vi "startService.vi"(8 "error in (no error)":errorcluster, 11 "M1M3SAL in":refnum<class "M1M3SAL.lvclass">) -> (0 "error out":errorcluster, 3 "M1M3SAL out":refnum<class "M1M3SAL.lvclass">)   [LabVIEW 2016, in "M1M3SupportCommunicator.lvlib" / "M1M3SAL.lvclass"]
uses:
  M1M3SAL.lvclass
  M1M3SAL.lvclass/M1M3SAL.ctl
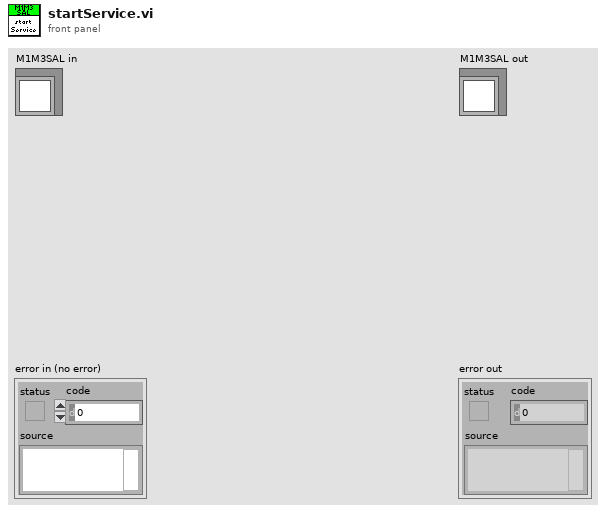
[diagram p1: front panel]
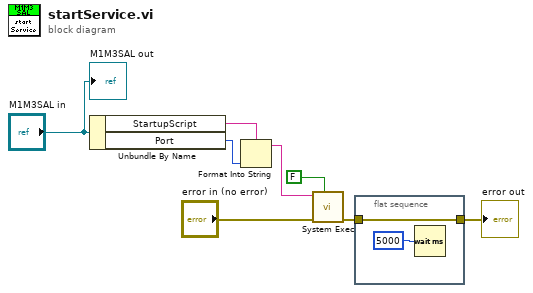
[diagram p0: block diagram]
diagram:
  n1 = Unbundle By Name("M1M3SAL in") -> ("StartupScript"=w8:string, "Port"=w7:u16)
  n2 = Format Into String(format string=w8, w7) -> (resulting string=w5:string)  [unwired: 2 in, 1 out]
  n3 = call <vilib>:"System Exec.vi"("wait until completion? (T)"=FALSE, "error in (no error)"="error in (no error)", "command line"=w5) -> ("error out"=w1:errorcluster)  [unwired: 5 in, 3 out]
  n4 = flat-sequence {
    tunnel: [w9] -> w2
    tunnel: w1 -> [w9]
    frame #0 {
      n5 = Wait (ms)(milliseconds to wait=u32 5000) -> ()  [unwired: 1 out]
    }
  }
  "error out" <- w2
  "M1M3SAL out" <- "M1M3SAL in"
